vi "SVT UFF58 Read Generic.vi"(0 "function refnum":refnum<k20>, 11 "error in (no error)":errorcluster) -> (3 "ID lines (1-3)":T1, 4 "dup function refnum":refnum<k20>, 6 "abscissa values (X)":dbl[](array[numeric]), 8 "ordinate values (Y Real)":dbl[](array[numeric]), 10 "ordinate values (Y Im)":dbl[](array[numeric]), 13 "abscissa minimum (x0)":dbl, 14 "abscissa increment (dx)":dbl, 15 "error out":errorcluster)   [LabVIEW 2017, in "SoundVib_UFF58.lvlib"]
doc: "Reads data from a UFF58 (universal file format) function specified by the <B>function refnum</B> input. This VI also reads the fields in records 1, 2, and 3, returned by ID lines (1-3). You can read a single time domain waveform, a single frequency spectrum, the real and imaginary parts of a frequency spectrum, and any data from a function. The default instance, SVT UFF58 Read Time Waveform, reads a single time domain waveform from a function specified by the <B>function refnum</B> input. Wire data to the <B>function refnum</B> input to determine the polymorphic instance to use or manually select the instance."
uses:
  <vilib>/addons/Sound and Vibration/svt_UFF58/SoundVib_UFF58.lvlib
  <vilib>/addons/Sound and Vibration/svt_UFF58/subVIs/sv_IDLines123.ctl
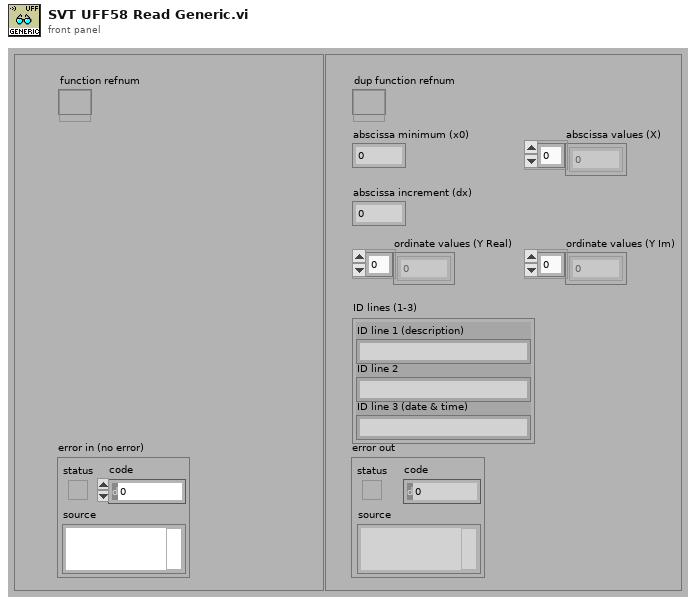
[diagram p1: front panel]
types:
  T1 = typedef "SoundVib_UFF58.lvlib/sv_IDLines123.ctl" = cluster{"ID line 1 (description)":string, "ID line 2":string, "ID line 3 (date & time)":string}
  T2 = typedef "SoundVib_UFF58.lvlib/sv_UFF58 Data Form.ctl" = cluster{"ordinate data type":u16, "number of data values/pairs":i32, "abscissa spacing":enum16{"uneven", "even"}, "abscissa minimum":dbl, "abscissa increment":dbl}
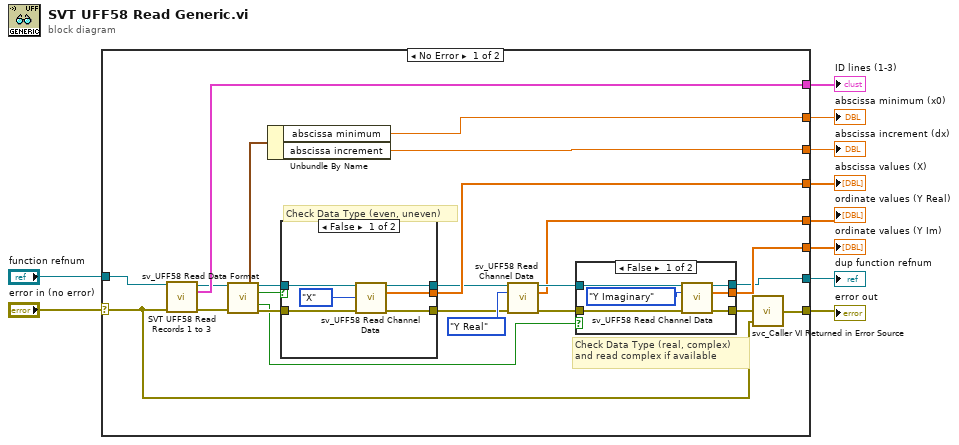
[diagram p0: block diagram]
diagram:
  n1 = case shown="No Error" "error in (no error)" {
    selector: "error in (no error)" -> [w14 w51]
    tunnel: [w30 _] -> w10
    tunnel: [w29 _] -> w9
    tunnel: [w28 _] -> w8
    tunnel: [w12 _] -> w7
    tunnel: [w11 _] -> w6
    tunnel: [w21 _] -> w5
    tunnel: [w20 w50] -> w1
    tunnel: [w15 w51] -> w4
    tunnel: "function refnum" -> [w17 w50]
    frame No Error {
      # "Check Data Type (real, complex) \nand read complex if available"
      # "Check Data Type (even, uneven)"
      n2 = call <vilib>:"SVT UFF58 Read Records 1 to 3.vi"("function refnum"=w17, "error in (no error)"=w14) -> ("dup function refnum"=w18:refnum<k20>, "ID lines (1-3)"=w21:T1, "error out"=w19:errorcluster)  [unwired: 11 in]
      n3 = call <vilib>:"sv_UFF58 Read Data Format.vi"("function refnum"=w18, "error in (no error)"=w19) -> ("data form"=w13:T2, "dup function refnum"=w27:refnum<k20>, "even"=w23:bool, "real"=w22:bool, "error out"=w26:errorcluster)  [unwired: 9 in]
      n4 = Unbundle By Name(w13) -> ("abscissa minimum"=w12:dbl, "abscissa increment"=w11:dbl)
      n5 = case shown="False" w23 {
        tunnel: [w43 _] -> w30
        tunnel: w27 -> [w47 w49]
        tunnel: w26 -> [w46 w48]
        tunnel: [w44 w49] -> w25
        tunnel: [w42 w48] -> w24
        frame False {
          n6 = call <vilib>:"sv_UFF58 Read Channel Data.vi"("function refnum"=w47, "channel to read"=enum16{"X", "Y Real", "Y Imaginary"}."X" ("data to read"), "error in (no error)"=w46) -> ("dup function refnum"=w44:refnum<k20>, "data"=w43:dbl[], "error out"=w42:errorcluster)  [unwired: 10 in]
        }
        frame True {
        }
      }
      n7 = call <vilib>:"sv_UFF58 Read Channel Data.vi"("function refnum"=w25, "channel to read"=enum16{"X", "Y Real", "Y Imaginary"}."Y Real" ("data to read"), "error in (no error)"=w24) -> ("dup function refnum"=w32:refnum<k20>, "data"=w28:dbl[], "error out"=w31:errorcluster)  [unwired: 10 in]
      n8 = case shown="False" w22 {
        tunnel: w31 -> [w39 w40]
        tunnel: w32 -> [w38 w41]
        tunnel: [w36 _] -> w29
        tunnel: [w35 w41] -> w20
        tunnel: [w34 w40] -> w16
        frame False {
          n9 = call <vilib>:"sv_UFF58 Read Channel Data.vi"("function refnum"=w38, "channel to read"=enum16{"X", "Y Real", "Y Imaginary"}."Y Imaginary" ("data to read"), "error in (no error)"=w39) -> ("dup function refnum"=w35:refnum<k20>, "data"=w36:dbl[], "error out"=w34:errorcluster)  [unwired: 10 in]
        }
        frame True {
        }
      }
      n10 = call <vilib>:"svc_Caller VI Returned in Error Source.vi"("warning input to caller"=w14, "error in (no error)"=w16) -> ("error out"=w15:errorcluster)  [unwired: 3 in]
    }
    frame Error {
    }
  }
  "error out" <- w4
  "abscissa values (X)" <- w10
  "ordinate values (Y Real)" <- w8
  "ordinate values (Y Im)" <- w9
  "abscissa minimum (x0)" <- w7
  "abscissa increment (dx)" <- w6
  "ID lines (1-3)" <- w5
  "dup function refnum" <- w1
